vi "AssignSetPressures.vi"(7 "Cal Ref":T1, 8 "Possible Water Mix Ratios":dbl[](array[numeric]), 9 "New Set Pressures":dbl[](array[numeric]), 10 "Set Water Mix Pressures In":dbl[](array[numeric]), 11 "Set Odor Pressures In":dbl[](array[numeric])) -> (2 "Set Water Mix Pressures":dbl[](array[numeric]), 3 "Set Odor Pressures":dbl[](array[numeric]))   [LabVIEW 2016]
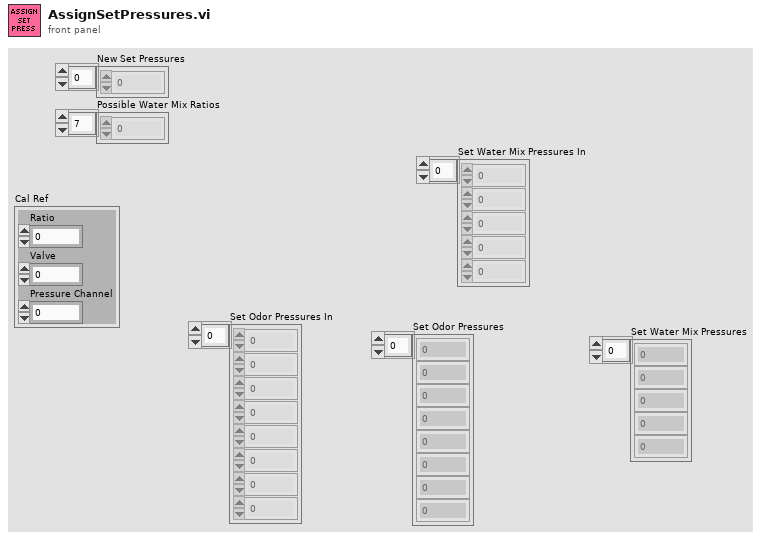
[diagram p1: front panel]
types:
  T1 = cluster{"Ratio":dbl, "Valve":u16, "Pressure Channel":u8}
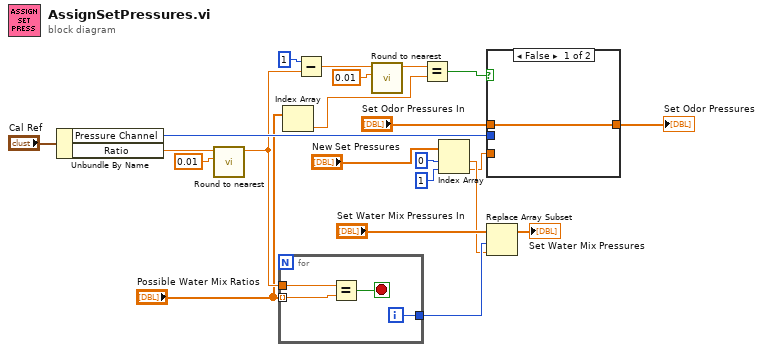
[diagram p0: block diagram]
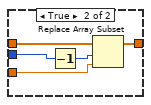
[diagram p2: hidden frame]
diagram:
  n1 = Unbundle By Name("Cal Ref") -> ("Pressure Channel"=w11:u8, "Ratio"=w21:dbl)
  n2 = call "Round to nearest.vi"("Round to nearest"=0.01, "Number"=w21) -> ("Rounded"=w7:dbl)  [unwired: 9 in]
  n3 = for {
    tunnel: w7 -> [w26]
    tunnel: "Possible Water Mix Ratios" -> [w25] mode=indexing
    tunnel: [w23] -> w19
    i -> [w23]
    stop <- w24 stop-if-true
    n4 = Equal?(x=w26, y=w25) -> (x = y?=w24:bool)
  }
  n5 = Index Array(array="Possible Water Mix Ratios") -> (element=w2:dbl)  [unwired: 1 in]
  n6 = Subtract(x=1, y=w7) -> (x-y=w6:dbl)
  n7 = call "Round to nearest.vi"("Round to nearest"=0.01, "Number"=w6) -> ("Rounded"=w4:dbl)  [unwired: 9 in]
  n8 = Equal?(x=w4, y=w2) -> (x = y?=w1:bool)
  n9 = Index Array(array="New Set Pressures", index #1=0 ("index"), index #2=1 ("index")) -> (element #1=w13:dbl, element #2=w12:dbl)
  n10 = case shown="False" w1 {
    tunnel: "Set Odor Pressures In" -> [w27 w32]
    tunnel: w12 -> [_ w31]
    tunnel: w11 -> [_ w30]
    tunnel: [w27 w28] -> w10
    frame False {
    }
    frame True {
      n11 = Decrement(x=w30) -> (x-1=w29:u8)
      n12 = Replace Array Subset(array=w32, new element=w31, index=w29) -> (w28:dbl[])
    }
  }
  "Set Odor Pressures" <- w10
  n13 = Replace Array Subset(array="Set Water Mix Pressures In", new element=w13, index=w19) -> (→"Set Water Mix Pressures":dbl[])
